vi "Fetch Waveform.vi"(8 "error in (no error)":errorcluster, 11 "Tektronix TDS 200 1000 2000 in":refnum<class "Tektronix TDS 200 1000 2000.lvclass">) -> (0 "error out":errorcluster, 2 "Waveform Data":waveform(dbl)[](graph), 3 "Tektronix TDS 200 1000 2000 out":refnum<class "Tektronix TDS 200 1000 2000.lvclass">)   [LabVIEW 2020, in "Tektronix TDS 200 1000 2000.lvclass"]
uses:
  Tektronix TDS 200 1000 2000.lvclass
  C:/Sandbox/Git_Sandbox/WiSpry Test Framework source code (LV20)/WiSpry Test Framework/Instruments/Instrument.lvclass
  Instrument.lvclass/Instrument.ctl
  Instrument.lvclass
  <instrlib>/Tektronix TDS 200 1000 2000 Series/Tektronix TDS 200 1000 2000 Series.lvlib
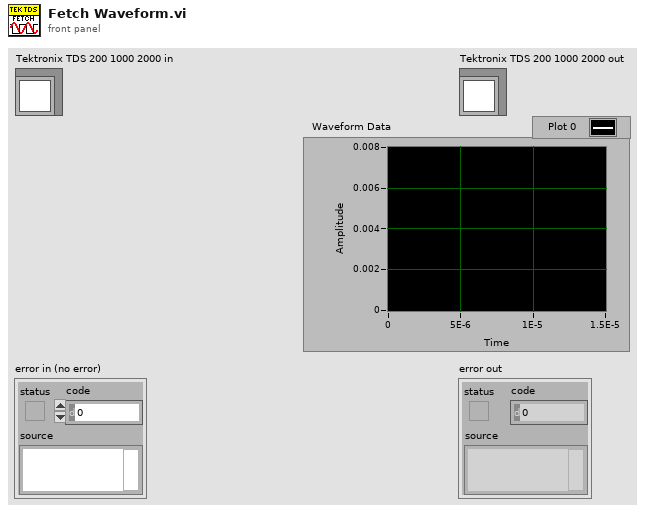
[diagram p1: front panel]
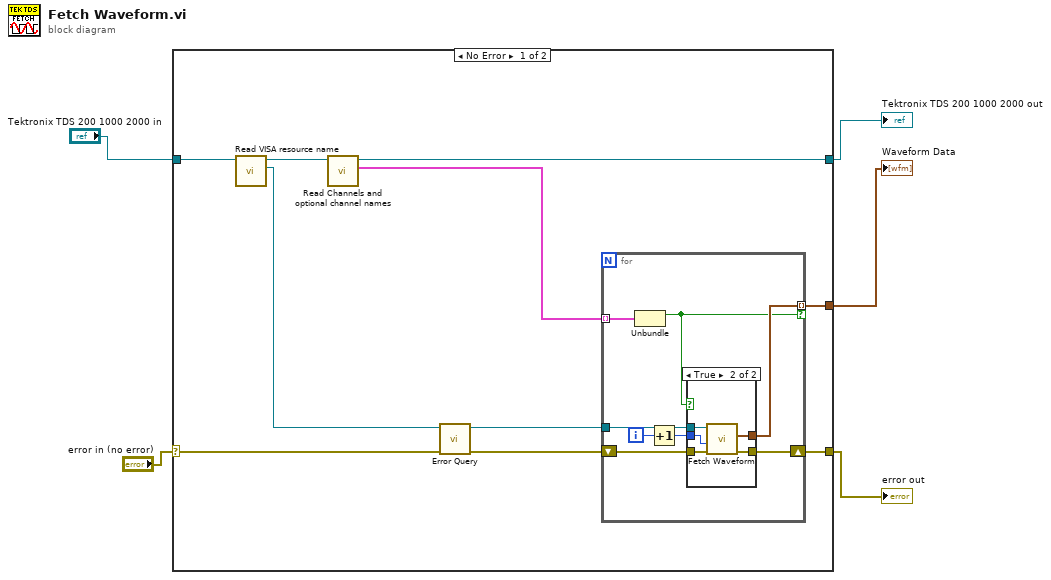
[diagram p0: block diagram]
diagram:
  n1 = case shown="No Error" "error in (no error)" {
    selector: "error in (no error)" -> [w9 w31]
    tunnel: [w10 w31] -> w1
    tunnel: [w13 w30] -> w3
    tunnel: "Tektronix TDS 200 1000 2000 in" -> [w15 w30]
    tunnel: [w11 _] -> w2
    frame No Error {
      n2 = call "Read VISA resource name.vi"("Instrument in"=w15) -> ("VISA resource name"=w6:refnum<visa-resource-name>, "Instrument out"=w14:refnum<class "Tektronix TDS 200 1000 2000.lvclass">)  [unwired: 9 in]
      n3 = call-dynamic "Read Channels and optional channel names.vi"("Oscilloscope in"=w14) -> ("Channels and optional channel names"=w12:cluster{"Enabled":bool, "Channel name":string}[], "Oscilloscope out"=w13:refnum<class "Tektronix TDS 200 1000 2000.lvclass">)  [unwired: 9 in]
      n4 = call <instrlib>:"Error Query.vi"("error in (no error)"=w9, "VISA resource name"=w6) -> ("error out"=w7:errorcluster, "VISA resource name out"=w8:refnum<visa-resource-name>)  [unwired: 6 in, 2 out]
      n5 = for {
        tunnel: w12 -> [w23] mode=indexing
        shift-right: [w19] -> w10
        shift-left: w7 -> [w21]
        tunnel: w8 -> [w20]
        tunnel: [w18] -> w11 mode=indexing if=w16
        i -> [w22]
        n6 = Unbundle(w23) -> ("Enabled"=w16:bool)  [unwired: 1 out]
        n7 = Increment(x=w22) -> (x+1=w17:i32)
        n8 = case shown="True" w16 {
          tunnel: w21 -> [w24 w29]
          tunnel: w20 -> [_ w28]
          tunnel: [w24 w27] -> w19
          tunnel: [_ w26] -> w18
          tunnel: w17 -> [_ w25]
          frame False {
          }
          frame True {
            n9 = call <instrlib>:"Fetch Waveform.vi"("error in (no error)"=w29, "Timeout (10000 ms)"=w25, "VISA resource name"=w28) -> ("error out"=w27:errorcluster, "Waveform Data"=w26:waveform(dbl))  [unwired: 6 in, 1 out]
          }
        }
      }
    }
    frame Error {
    }
  }
  "error out" <- w1
  "Tektronix TDS 200 1000 2000 out" <- w3
  "Waveform Data" <- w2
